vi "ReturnToJoystick.vi"   [LabVIEW 2020]
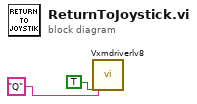
[diagram p0: block diagram]
diagram:
  n1 = call "Vxmdriverlv8.Vi"("Send\nchars\nto port"=TRUE, "Chars to send"="Q" ("string")) -> ()  [unwired: 20 in, 6 out]
